vi "Dashboard Main.vi"() -> ()   [LabVIEW 2013]
uses:
  Robot Code - Final/2014 Target Detection/TargetType.ctl
  <vilib>/event_ctls.llb/eventvkey.ctl
  <vilib>/Rock Robotics/WPI/Dashboard/WPI_DashboardLogging Global.vi
  <vilib>/Utility/config.llb/Write Key (String).vi
  <vilib>/Utility/config.llb/Write Key (I32).vi
  <vilib>/Utility/config.llb/NI_LVConfig.lvlib
panel:
  in  "Camera Type":enum16{"206", "1011", "1013"}(ring)=enum."1013"
  out "Image Message":string="Timeout in Camera Communications"
  in  "Rec Mode":enum32{"Stop", "Record", "Playback"}(radio)
  in  "Dashboard Tab":T1(tab)
  in  "X-box":bool caption="Joystick"
  out "Speed (RPM x1000)":dbl(knob) scale=0.0..6.0
  out "Bag Motors":dbl(knob) scale=-1.0..1.0
  out "ENG":bool
  out "DIS":bool
  out "Pickup":dbl(knob) scale=-1.0..1.0 scale format="%#_1g"
  out "Fire":bool
  out "Pick up":bool
  out "Shooter":bool
  in  "Camera Settings":T2={"Frame Rate"=30, "Compression"=30, "Size"=1} {"Frame Rate" scale=1.0..30.0; "Size" items=["640x480", "320x240", "160x120"]}
  out "MotorSliders R":cluster{"MotorSlide1":dbl, "MotorSlide2":dbl} {"MotorSlide2" scale=-1.0..1.0 scale format="%#_2e"; "MotorSlide1" scale=-1.0..1.0 scale format="%#_2e"}
  out "MotorChart R":cluster{"Numeric":dbl, "Numeric":dbl}(graph)
  out "MotorSliders L":T3 {"MotorSlide4 2" scale=0.0..14.0 scale format="%#_2e"; "MotorSlide2" scale=-1.0..1.0 scale format="%#_2e"; "MotorSlide1" scale=-1.0..1.0 scale format="%#_2e"}
  out "MotorChart L":T4(graph)
  out "JS1 Z":dbl(slide) scale=-1.0..1.0 scale format="%#_2e"
  out "Joystick 1":cluster{"X":dbl, "Y":dbl}[](graph)
  out "JS Buttons 1":T5
  out "JS2 Z":dbl(slide) scale=-1.0..1.0 scale format="%#_2e"
  out "Joystick 2":cluster{"X":dbl, "Y":dbl}[](graph)
  out "JS Buttons 2":T5
  out "Mode":T6(ring)=enum."Auto Disabled"
  out "Camera IP":string
  in  "DB Camera Config":bool
  out "fps":dbl format="%#.1g"
  out "Mbps":dbl format="%#.1g"
  out "Mbps 2":bool
  out "LED 1":bool
  in  "Score Limit":dbl=70.0
  out "Distance":dbl
  out "Target Locked On":bool
  in  "Slider 1":dbl(slide) scale=0.0..100.0
  out "Goal is hot":bool
  out "Distances":T8(array[cluster])
  in  "Color Components":T9={"Hue"={110.0, 142.0}, "Sat"={138.0, 255.0}, "Val"={139.0, 198.0}} {"Val" scale=0.0..255.0; "Sat" scale=0.0..255.0; "Hue" scale=0.0..255.0 scale format="%#_3g"}
  in  "Checkbox 2":bool
  in  "Checkbox 1":bool
  in  "Test Slider":dbl(slide) scale=0.0..100.0 scale format="%#_3g"
  in  "On/Off":bool caption="Solenoid"
  in  "Test Name":u16(ring) items=["Select the test to run...", "Example Test", "-------------------------------", "List of tests is built in robot code.", "Replace with your own automated tests."]
  in  "Test Tree":string(tree)
  in  "Motor":cluster{"Value":dbl, "Enable":bool} {"Value" scale=-1.0..1.0 scale format="%#_3g"}
  out "Progress":T10 {"Test Progress" scale=0.0..100.0}
  in  "Rev/Fwd":cluster{"Forward":bool, "Reverse":bool}
  in  "Test Ring":u16(ring) items=["Auto", "Fixed indoor", "Fixed outdoor 1", "Fixed outdoor 2", "Fixed fluorescent 1", "Fixed fluorescent 2", "Hold current"]
  in  "Listbox":i32(listbox)
  out "Tree":string(tree)
  out "Camera Image":T11(plugin-control)
  in  "Enable":bool
  # "Left"
  # "Front"
  # "Right"
  # "Gearbox"
  # "Battery"
  # "Customize by placing controls and indicators here and name to\nmatch Dashboard Variables on robot."
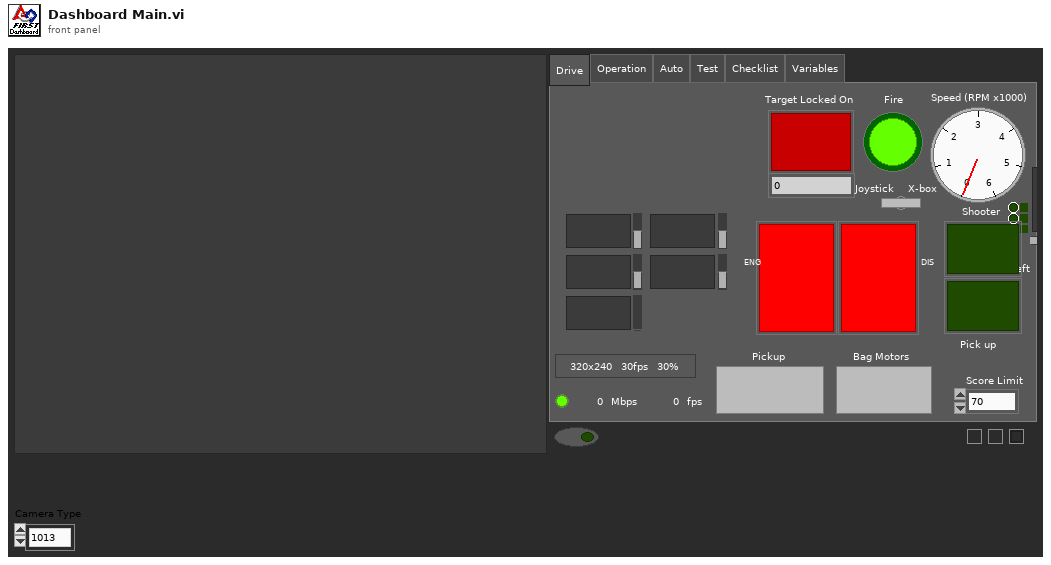
[diagram p1: front panel]
types:
  T1 = enum32{"Drive", "Operation", "Auto", "Test", "Checklist", "Variables"}
  T2 = cluster{"Frame Rate":i32, "Compression":i32, "Size":u16}
  T3 = cluster{"MotorSlide1":dbl, "MotorSlide2":dbl, "MotorSlide4 2":dbl}
  T4 = cluster{"Numeric":dbl, "Numeric":dbl, "Battery":sgl}
  T5 = cluster{bool, bool, bool, bool, bool, bool, bool, bool, bool, bool, bool, bool}
  T6 = enum8{"Tele-Op Disabled", "Tele-Op Enabled", "Auto Disabled", "Auto Enabled", "Test Disabled", "Test Enabled", ""}
  T7 = typedef "TargetType.ctl" = enum16{"Not Hot", "Hot"}
  T8 = cluster{"Distance (ft)":dbl, "Target Center (-1 to 1)":cluster{"X":dbl, "Y":dbl}, "Left":bool, "State":T7}[]
  T9 = cluster{"Hue":cluster{dbl, dbl}, "Sat":cluster{dbl, dbl}, "Val":cluster{dbl, dbl}}
  T10 = cluster{"Test Progress":u8, "Test Progress Text":string}
  T11 = typedef "IMAQ Image.ctl" = refnum<image>
  T12 = typedef "Image Type" = u32
  T13 = cluster{"Digital Inputs":bool[], "Digital Outputs":bool[]}
  T14 = cluster{"Competition mode":bool, "Robot Link":bool, "Autonomous":bool, "Enabled":bool, "E-Stop":bool, "Simulated":bool, "TestMode":bool, "Docked Window":bool}
  T15 = cluster{"Boolean Array[0]":bool, "Boolean Array[1]":bool, "Boolean Array[2]":bool, "Boolean Array[3]":bool, "Boolean Array[4]":bool, "Boolean Array[5]":bool, "Boolean Array[6]":bool, "Boolean Array[7]":bool, "Boolean Array[8]":bool, "Boolean Array[9]":bool, "Boolean Array[10]":bool, "Boolean Array[11]":bool}
  T16 = cluster{"Horizontal":bool, "Aspect Score":dbl, "Rect Score":dbl, cluster{"Left":dbl, "Top":dbl, "Right":dbl, "Bottom":dbl}, "Equiv H":dbl, "Equiv V":dbl}[]
  T17 = cluster{"Scores":cluster{"Total":dbl, "Left":dbl, "Right":dbl, "Ratio":dbl, "Vertical":dbl, "index":i32, "State":T7}, "Verticals":cluster{"Horizontal?":bool, "Aspect Score":dbl, "Rect Score":dbl, cluster{"Left":dbl, "Top":dbl, "Right":dbl, "Bottom":dbl}, "Equiv H":dbl, "Equiv V":dbl}, "Horizontals":cluster{"Horizontal?":bool, "Aspect Score":dbl, "Rect Score":dbl, cluster{"Left":dbl, "Top":dbl, "Right":dbl, "Bottom":dbl}, "Equiv H":dbl, "Equiv V":dbl}, "Validated":bool}[]
  T18 = cluster{"Scores":cluster{"Total":dbl, "Left":dbl, "Right":dbl, "Ratio":dbl, "Vertical":dbl, "index":i32, "State":T7}, "Verticals":cluster{"Horizontal?":bool, "Aspect Score":dbl, "Rect Score":dbl, cluster{"Left":dbl, "Top":dbl, "Right":dbl, "Bottom":dbl}, "Equiv H":dbl, "Equiv V":dbl}, "Horizontals":cluster{"Horizontal?":bool, "Aspect Score":dbl, "Rect Score":dbl, cluster{"Left":dbl, "Top":dbl, "Right":dbl, "Bottom":dbl}, "Equiv H":dbl, "Equiv V":dbl}, "Distance (ft)":dbl, "Target Center (-1 to 1)":cluster{"X":dbl, "Y":dbl}}[]
  T19 = cluster{"Target Info[0]":cluster{"Scores":cluster{"Total":dbl, "Left":dbl, "Right":dbl, "Ratio":dbl, "Vertical":dbl, "index":i32, "State":T7}, "Verticals":cluster{"Horizontal?":bool, "Aspect Score":dbl, "Rect Score":dbl, cluster{"Left":dbl, "Top":dbl, "Right":dbl, "Bottom":dbl}, "Equiv H":dbl, "Equiv V":dbl}, "Horizontals":cluster{"Horizontal?":bool, "Aspect Score":dbl, "Rect Score":dbl, cluster{"Left":dbl, "Top":dbl, "Right":dbl, "Bottom":dbl}, "Equiv H":dbl, "Equiv V":dbl}, "Distance (ft)":dbl, "Target Center (-1 to 1)":cluster{"X":dbl, "Y":dbl}}, "Target Info[1]":cluster{"Scores":cluster{"Total":dbl, "Left":dbl, "Right":dbl, "Ratio":dbl, "Vertical":dbl, "index":i32, "State":T7}, "Verticals":cluster{"Horizontal?":bool, "Aspect Score":dbl, "Rect Score":dbl, cluster{"Left":dbl, "Top":dbl, "Right":dbl, "Bottom":dbl}, "Equiv H":dbl, "Equiv V":dbl}, "Horizontals":cluster{"Horizontal?":bool, "Aspect Score":dbl, "Rect Score":dbl, cluster{"Left":dbl, "Top":dbl, "Right":dbl, "Bottom":dbl}, "Equiv H":dbl, "Equiv V":dbl}, "Distance (ft)":dbl, "Target Center (-1 to 1)":cluster{"X":dbl, "Y":dbl}}, "Target Info[2]":cluster{"Scores":cluster{"Total":dbl, "Left":dbl, "Right":dbl, "Ratio":dbl, "Vertical":dbl, "index":i32, "State":T7}, "Verticals":cluster{"Horizontal?":bool, "Aspect Score":dbl, "Rect Score":dbl, cluster{"Left":dbl, "Top":dbl, "Right":dbl, "Bottom":dbl}, "Equiv H":dbl, "Equiv V":dbl}, "Horizontals":cluster{"Horizontal?":bool, "Aspect Score":dbl, "Rect Score":dbl, cluster{"Left":dbl, "Top":dbl, "Right":dbl, "Bottom":dbl}, "Equiv H":dbl, "Equiv V":dbl}, "Distance (ft)":dbl, "Target Center (-1 to 1)":cluster{"X":dbl, "Y":dbl}}, "Target Info[3]":cluster{"Scores":cluster{"Total":dbl, "Left":dbl, "Right":dbl, "Ratio":dbl, "Vertical":dbl, "index":i32, "State":T7}, "Verticals":cluster{"Horizontal?":bool, "Aspect Score":dbl, "Rect Score":dbl, cluster{"Left":dbl, "Top":dbl, "Right":dbl, "Bottom":dbl}, "Equiv H":dbl, "Equiv V":dbl}, "Horizontals":cluster{"Horizontal?":bool, "Aspect Score":dbl, "Rect Score":dbl, cluster{"Left":dbl, "Top":dbl, "Right":dbl, "Bottom":dbl}, "Equiv H":dbl, "Equiv V":dbl}, "Distance (ft)":dbl, "Target Center (-1 to 1)":cluster{"X":dbl, "Y":dbl}}, "Target Info[4]":cluster{"Scores":cluster{"Total":dbl, "Left":dbl, "Right":dbl, "Ratio":dbl, "Vertical":dbl, "index":i32, "State":T7}, "Verticals":cluster{"Horizontal?":bool, "Aspect Score":dbl, "Rect Score":dbl, cluster{"Left":dbl, "Top":dbl, "Right":dbl, "Bottom":dbl}, "Equiv H":dbl, "Equiv V":dbl}, "Horizontals":cluster{"Horizontal?":bool, "Aspect Score":dbl, "Rect Score":dbl, cluster{"Left":dbl, "Top":dbl, "Right":dbl, "Bottom":dbl}, "Equiv H":dbl, "Equiv V":dbl}, "Distance (ft)":dbl, "Target Center (-1 to 1)":cluster{"X":dbl, "Y":dbl}}, "Target Info[5]":cluster{"Scores":cluster{"Total":dbl, "Left":dbl, "Right":dbl, "Ratio":dbl, "Vertical":dbl, "index":i32, "State":T7}, "Verticals":cluster{"Horizontal?":bool, "Aspect Score":dbl, "Rect Score":dbl, cluster{"Left":dbl, "Top":dbl, "Right":dbl, "Bottom":dbl}, "Equiv H":dbl, "Equiv V":dbl}, "Horizontals":cluster{"Horizontal?":bool, "Aspect Score":dbl, "Rect Score":dbl, cluster{"Left":dbl, "Top":dbl, "Right":dbl, "Bottom":dbl}, "Equiv H":dbl, "Equiv V":dbl}, "Distance (ft)":dbl, "Target Center (-1 to 1)":cluster{"X":dbl, "Y":dbl}}, "Target Info[6]":cluster{"Scores":cluster{"Total":dbl, "Left":dbl, "Right":dbl, "Ratio":dbl, "Vertical":dbl, "index":i32, "State":T7}, "Verticals":cluster{"Horizontal?":bool, "Aspect Score":dbl, "Rect Score":dbl, cluster{"Left":dbl, "Top":dbl, "Right":dbl, "Bottom":dbl}, "Equiv H":dbl, "Equiv V":dbl}, "Horizontals":cluster{"Horizontal?":bool, "Aspect Score":dbl, "Rect Score":dbl, cluster{"Left":dbl, "Top":dbl, "Right":dbl, "Bottom":dbl}, "Equiv H":dbl, "Equiv V":dbl}, "Distance (ft)":dbl, "Target Center (-1 to 1)":cluster{"X":dbl, "Y":dbl}}, "Target Info[7]":cluster{"Scores":cluster{"Total":dbl, "Left":dbl, "Right":dbl, "Ratio":dbl, "Vertical":dbl, "index":i32, "State":T7}, "Verticals":cluster{"Horizontal?":bool, "Aspect Score":dbl, "Rect Score":dbl, cluster{"Left":dbl, "Top":dbl, "Right":dbl, "Bottom":dbl}, "Equiv H":dbl, "Equiv V":dbl}, "Horizontals":cluster{"Horizontal?":bool, "Aspect Score":dbl, "Rect Score":dbl, cluster{"Left":dbl, "Top":dbl, "Right":dbl, "Bottom":dbl}, "Equiv H":dbl, "Equiv V":dbl}, "Distance (ft)":dbl, "Target Center (-1 to 1)":cluster{"X":dbl, "Y":dbl}}, "Target Info[8]":cluster{"Scores":cluster{"Total":dbl, "Left":dbl, "Right":dbl, "Ratio":dbl, "Vertical":dbl, "index":i32, "State":T7}, "Verticals":cluster{"Horizontal?":bool, "Aspect Score":dbl, "Rect Score":dbl, cluster{"Left":dbl, "Top":dbl, "Right":dbl, "Bottom":dbl}, "Equiv H":dbl, "Equiv V":dbl}, "Horizontals":cluster{"Horizontal?":bool, "Aspect Score":dbl, "Rect Score":dbl, cluster{"Left":dbl, "Top":dbl, "Right":dbl, "Bottom":dbl}, "Equiv H":dbl, "Equiv V":dbl}, "Distance (ft)":dbl, "Target Center (-1 to 1)":cluster{"X":dbl, "Y":dbl}}}
  T20 = cluster{cluster{dbl, dbl}, cluster{dbl, dbl}, cluster{dbl, dbl}}
  T21 = typedef "NI_LVConfig.lvlib/Config Data RefNum.ctl" = refnum<k1>
  T22 = typedef "eventvkey.ctl" = enum16{"ASCII", "Enter", "Return", "Shift", "Ctrl", "Alt", "Cmd", "Opt", "Caps", "NumLock", "Clear", "Break", "Up", "Down", "Left", "Right", "Insert", "Delete", "Home", "End", "PageUp", "PageDown", "Escape", "Help", "Pause", "ScrollLock", "F1", "F2", "F3", "F4", "F5", "F6", "F7", "F8", "F9", "F10", "F11", "F12", "F13", "F14", "F15", "F16", "F17", "F18", "F19", "F20", "F21", "F22", "F23", "F24", "Play", "VolumeUp", "VolumeDown", "Mute", "Two Byte Char"}
  T23 = cluster{"Image Size":bool, "Image Type":bool, "Pixel Value":bool, "ROI Information":bool, "Zoom Factor":bool}
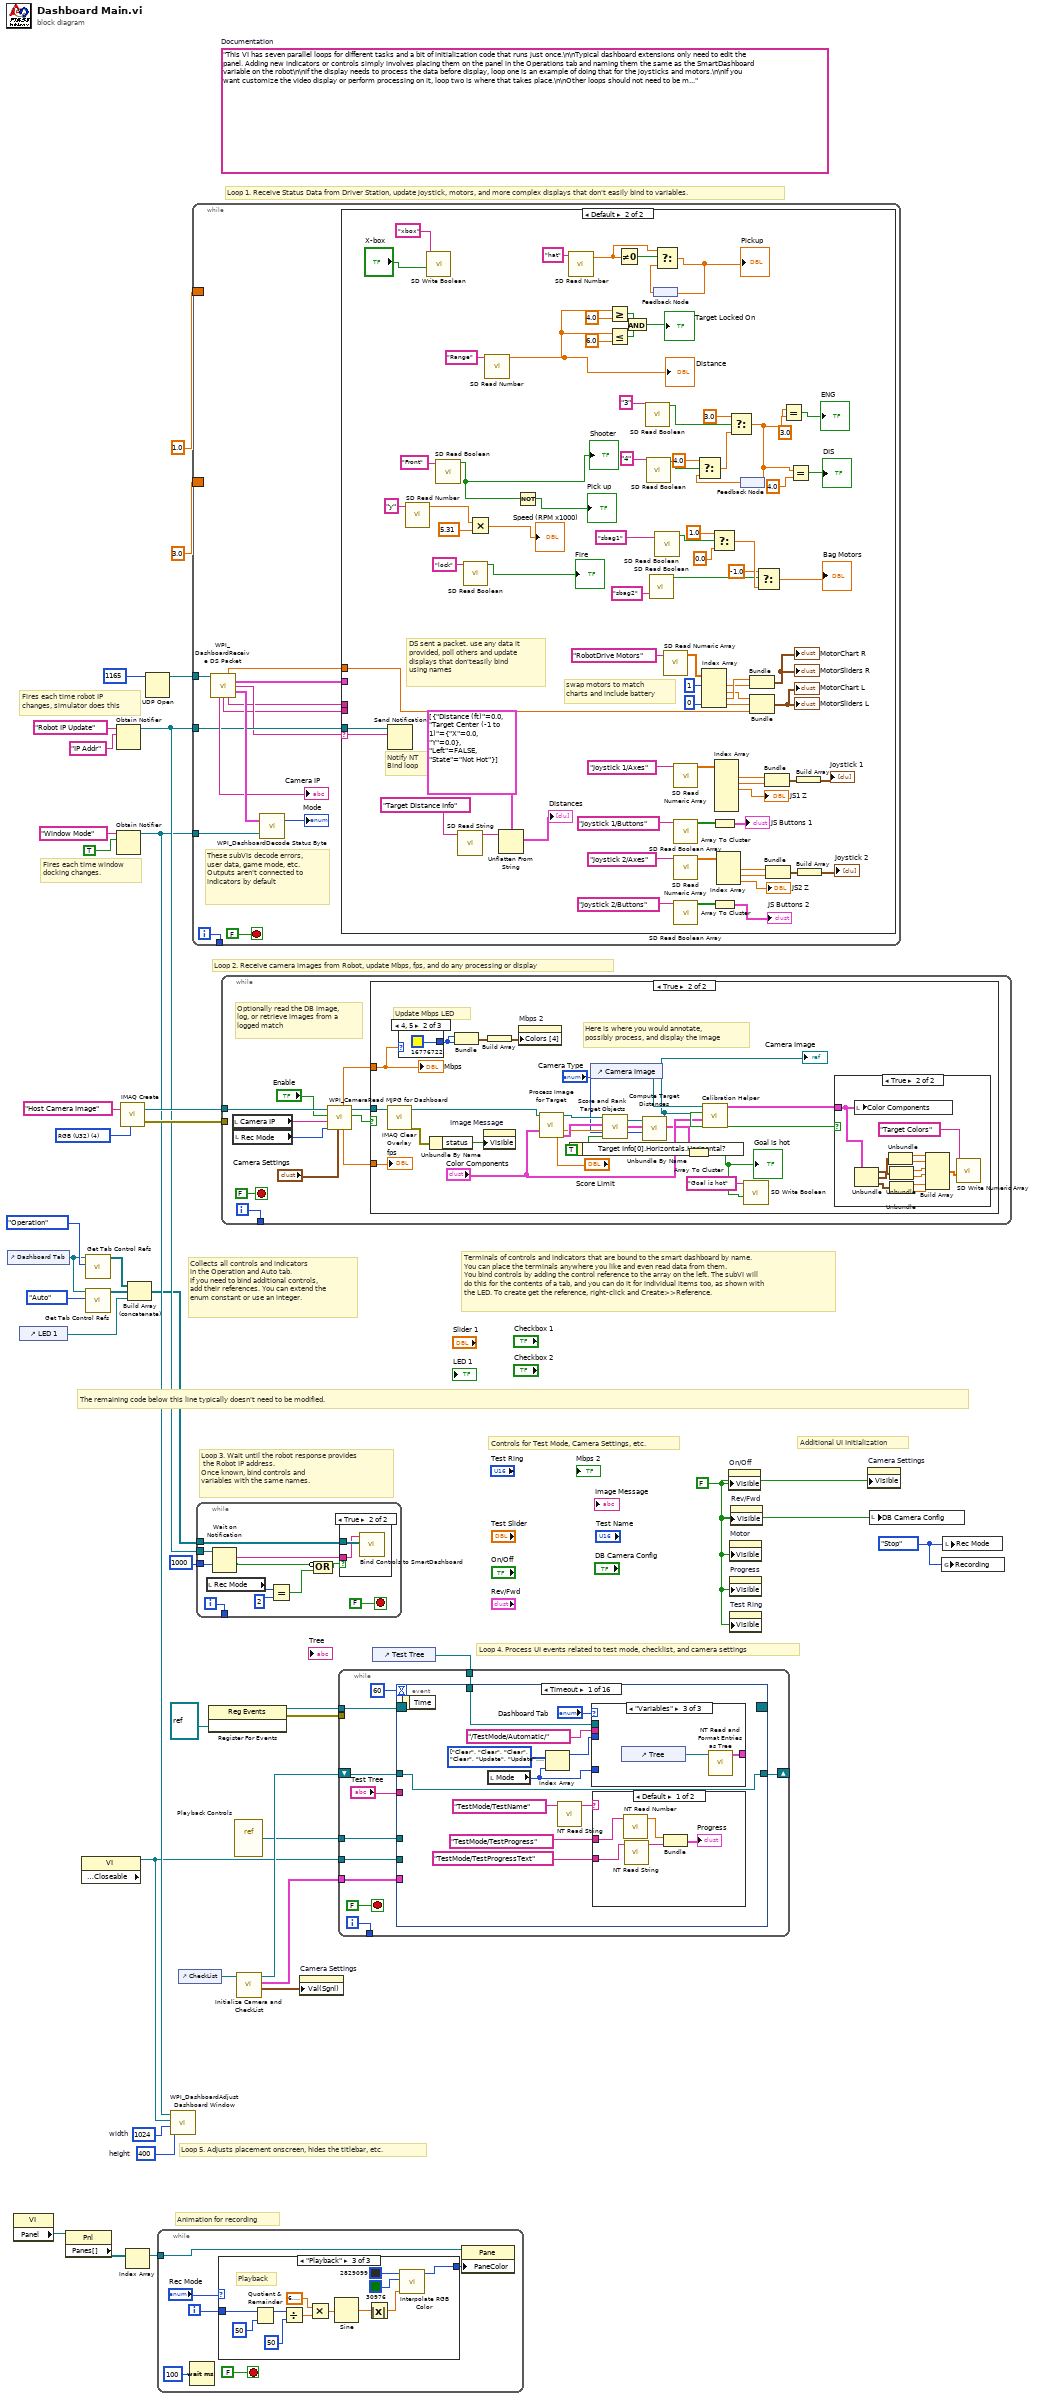
[diagram p0: block diagram]
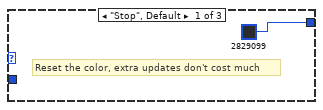
[diagram p2: hidden frame]
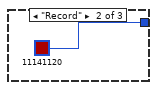
[diagram p3: hidden frame]
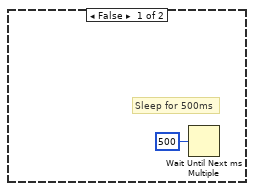
[diagram p5: hidden frame]
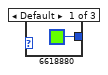
[diagram p7: hidden frame]
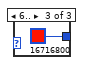
[diagram p8: hidden frame]
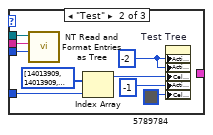
[diagram p10: hidden frame]
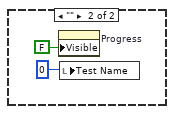
[diagram p11: hidden frame]
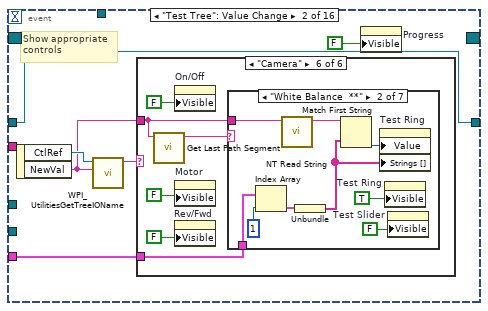
[diagram p12: hidden frame]
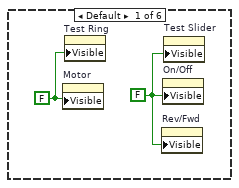
[diagram p13: hidden frame]
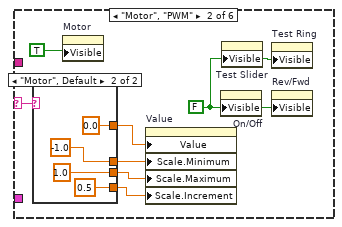
[diagram p14: hidden frame]
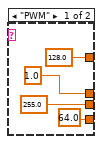
[diagram p15: hidden frame]
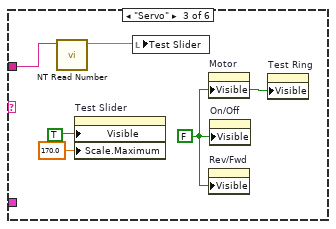
[diagram p16: hidden frame]
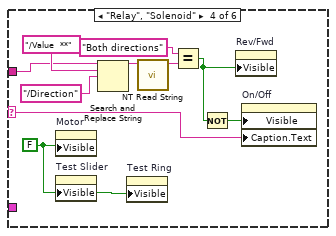
[diagram p17: hidden frame]
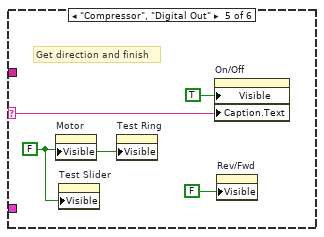
[diagram p18: hidden frame]
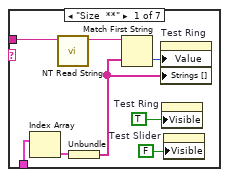
[diagram p19: hidden frame]
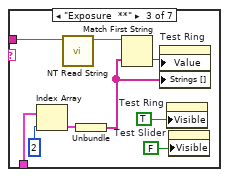
[diagram p20: hidden frame]
diagram:
  w10 = enum32{"Stop", "Record", "Playback"}."Stop" ("Rec Mode")
  w13 = 400  # height
  w14 = 1024  # width
  w27 = FALSE ("Visible")
  (unwired) "This VI has seven parallel loops for different tasks and a bit of initialization code that runs just once.\n\nTypical dashboard extensions only need to edit the panel. Adding new indicators or controls simply involves placing them on the panel in the Operations tab and naming them the same as the SmartDashboard variable on the robot\n\nIf the display needs to process the data before display, loop one is an example of doing that for the joysticks and motors.\n\nIf you want customize the video display or perform processing on it, loop two is where that takes place.\n\nOther loops should not need to be modified. They are pretty standard, and document the task they perform."  # Documentation
  w37 = T12 4 items=["Grayscale (U8)", "Grayscale (I16)", "Grayscale (SGL)", "Complex (CSG)", "RGB (U32)", "HSL (U32)", "RGB (U64)"] ("Image Type")
  # "Controls for Test Mode, Camera Settings, etc."
  # "Additional UI Initialization"
  # "Animation for recording"
  # "Fires each time robot IP\nchanges, simulator does this"
  # "Fires each time window\ndocking changes."
  # "Collects all controls and indicators\nin the Operation and Auto tab.\nIf you need to bind additional controls,\nadd their references. You can extend the\nenum constant or use an integer."
  # "The remaining code below this line typically doesn't need to be modified."
  # "Loop 4. Process UI events related to test mode, checklist, and camera settings"
  # "Terminals of controls and indicators that are bound to the smart dashboard by name.\nYou can place the terminals anywhere you like and even read data from them.\nYou bind controls by adding the control reference to the array on the left. The subVI will\ndo this for the contents of a tab, and you can do it for individual items too, as shown with\nthe LED. To create get the reference, right-click and Create>>Reference."
  # "Loop 3. Wait until the robot response provides\n the Robot IP address.\nOnce known, bind controls and\nvariables with the same names."
  # "Loop 5. Adjusts placement onscreen, hides the titlebar, etc."
  # "Loop 1. Receive Status Data from Driver Station, update joystick, motors, and more complex displays that don't easily bind to variables."
  # "Loop 2. Receive camera images from Robot, update Mbps, fps, and do any processing or display"
  n1 = control-ref of="Dashboard Tab"() -> (w8:refnum<vi>)
  n2 = property class="VI"() -> ("Panel"=w21:refnum<vi>)  [unwired: 2 in, 2 out]
  n3 = control-ref of="LED 1"() -> (w3:refnum<vi>)
  n4 = property class="Pnl"(reference=w21) -> ("Panes[]"=w22:refnum<vi>[])  [unwired: 1 in, 2 out]
  n5 = property class="VI" props=["Front Panel.Closeable"]() -> (reference out=w9:refnum<vi>)  [unwired: 2 in, 2 out]
  n6 = call <vilib>:"Get Tab Control Refs.vi"("Page Index"=T1."Operation" ("Dashboard Tab"), "TabControl in"=w8) -> ("ControlsOnPage"=w6:refnum<vi>[])  [unwired: 9 in]
  n7 = call <vilib>:"Get Tab Control Refs.vi"("Page Index"=T1."Auto" ("Dashboard Tab"), "TabControl in"=w8) -> ("ControlsOnPage"=w7:refnum<vi>[])  [unwired: 9 in]
  n8 = Obtain Notifier(name (unnamed)="Robot IP Update", notification data type="IP Addr" ("name (unnamed)")) -> (notifier out=w31:refnum<notifier>)  [unwired: 2 in, 2 out]
  n9 = Obtain Notifier(name (unnamed)="Window Mode", notification data type=TRUE) -> (notifier out=w12:refnum<notifier>)  [unwired: 2 in, 2 out]
  n10 = call "IMAQ Create"("Image Name"="Host Camera Image", "Image Type"=w37) -> ("New Image"=w35:T11, "error out"=w34:errorcluster)  [unwired: 2 in, 1 out]
  n11 = Index Array(array=w22) -> (element=w20:refnum<vi>)  [unwired: 1 in]
  n12 = Build Array (concatenate)(w6, w7, w3) -> (w5:refnum<vi>[])
  n13 = UDP Open(11:u16 1165 ("port")) -> (port=w38:refnum<k16>)  [unwired: 2 in, 4 out]
  n14 = while {
    tunnel: w20 -> [w41]
    i -> [w44]
    stop <- FALSE stop-if-true
    n15 = Wait (ms)(milliseconds to wait=u32 100) -> ()  [unwired: 1 out]
    n16 = case shown="\"Playback\"" "Rec Mode" {
      tunnel: w44 -> [_ _ w59]
      tunnel: [u32 2829099 ("Base Color") u32 11141120 ("Target Color") w48] -> w40
      frame "Stop", Default {
        # "Reset the color, extra updates don't cost much"
      }
      frame "Record" {
      }
      frame "Playback" {
        # "Playback"
        n17 = Quotient & Remainder(x=w59, y=u32 50 ("milliseconds to wait")) -> (x-y*floor(x/y)=w55:u32)  [unwired: 1 out]
        n18 = Divide(x=w55, y=u32 50 ("milliseconds to wait")) -> (x/y=w52:dbl)
        n19 = Multiply(x=6.283185307179586, y=w52) -> (x*y=w57:dbl)
        n20 = Sine(x=w57) -> (sin(x)=w56:dbl)
        n21 = Absolute Value(x=w56) -> (abs(x)=w49:dbl)
        n22 = call "Interpolate RGB Color.vi"("Proportion"=w49, "Target Color"=u32 30976, "Base Color"=u32 2829099) -> ("Result Color"=w48:u32)  [unwired: 8 in]
      }
    }
    n23 = property class="Pane"(reference=w41, "PaneColor"=w40) -> ()  [unwired: 1 in, 2 out]
  }
  n24 = call <vilib>:"WPI_DashboardAdjust Dashboard Window.vi"("height"=w13, "width"=w14, "reference in"=w9, "Notifier in"=w12) -> ()  [unwired: 8 in]
  n25 = control-ref of="CheckList"() -> (w11:refnum<vi>)
  n26 = while {
    tunnel: w38 -> [w70]
    tunnel: w31 -> [w65]
    tunnel: w12 -> [w69]
    tunnel: [w66] -> _
    border: 3.0 -> [_]
    border: 1.0 ("Numeric") -> [_]
    i -> [w66]
    stop <- FALSE stop-if-true
    # "These subVIs decode errors, user data, game mode, etc.\nOutputs aren't connected to indicators by default"
    n27 = call <vilib>:"WPI_DashboardReceive DS Packet.vi"("Recv Socket"=w70) -> ("Battery"=w60:sgl, "Driver Station"=w61:T13, "Robot IP Address"=w64:string, "Status"=w71:T14, "Camera IP Address"=→"Camera IP":string, "Low Priority User Data"=w63:string, "High Priority User Data"=w62:string)  [unwired: 1 in, 7 out]
    n28 = call <vilib>:"WPI_DashboardDecode Status Byte.vi"("Window Mode Notifier"=w69, "Status"=w71) -> ("Mode"=→"Mode":T6)  [unwired: 1 out]
    n29 = case shown="Default" w64 {
      selector: w64 -> [_ w132]
      tunnel: w65 -> [_ w133]
      tunnel: w63 -> [_ _]
      tunnel: w62 -> [_ _]
      tunnel: w61 -> [_ _]
      tunnel: w60 -> [_ w131]
      frame "0.0.0.0" {
        # "DS not sending packets, or no robot exists yet.\nDon't poll the variables"
      }
      frame Default {
        # "Notify NT\nBind loop"
        # "DS sent a packet. use any data it\nprovided, poll others and update\ndisplays that don'teasily bind\nusing names"
        # "swap motors to match\ncharts and include battery"
        n30 = Send Notification(notification=w132, notifier=w133) -> ()  [unwired: 1 in, 2 out]
        n31 = call <vilib>:"SD Read Number.vi"("Name"="y") -> ("Numeric"=w86:dbl)  [unwired: 8 in, 2 out]
        n32 = call <vilib>:"SD Write Boolean.vi"("Boolean"="X-box", "Name"="xbox") -> ()  [unwired: 8 in, 2 out]
        n33 = call <vilib>:"SD Read Boolean.vi"("Name"="Front") -> ("Boolean"=w88:bool)  [unwired: 8 in, 2 out]
        "Shooter" <- w88
        n34 = call <vilib>:"SD Read String.vi"("Name"="Target Distance Info") -> ("String"=w121:string)  [unwired: 8 in, 2 out]
        n35 = call <vilib>:"SD Read Boolean.vi"("Name"="lock") -> ("Boolean"=→"Fire":bool)  [unwired: 8 in, 2 out]
        n36 = Multiply(x=w86, y=5.31) -> (x*y=→"Speed (RPM x1000)":dbl)
        n37 = call <vilib>:"SD Read Number.vi"("Name"="Range") -> ("Numeric"=w116:dbl)  [unwired: 8 in, 2 out]
        "Distance" <- w116
        n38 = Unflatten From String(type=T8 [{"Distance (ft)"=0.0, "Target Center (-1 to 1)"={"X"=0.0, "Y"=0.0}, "Left"=FALSE, "State"=enum."Not Hot"}] ("Distances"), binary string=w121) -> (value=→"Distances":T8)  [unwired: 3 in, 2 out]
        n39 = Not(x=w88) -> (.not. x?=→"Pick up":bool)
        n40 = call <vilib>:"SD Read Number.vi"("Name"="hat") -> ("Numeric"=w92:dbl)  [unwired: 8 in, 2 out]
        n41 = Greater Or Equal?(x=w116, y=4.0) -> (x >= y?=w113:bool)
        n42 = Less Or Equal?(x=w116, y=6.0) -> (x <= y?=w112:bool)
        n43 = Not Equal To 0?(x=w92) -> (x != 0?=w93:bool)
        n44 = And(x=w113, y=w112) -> (x .and. y?=→"Target Locked On":bool)
        n45 = call <vilib>:"SD Read Boolean.vi"("Name"="3") -> ("Boolean"=w103:bool)  [unwired: 8 in, 2 out]
        n46 = call <vilib>:"SD Read Boolean.vi"("Name"="4") -> ("Boolean"=w104:bool)  [unwired: 8 in, 2 out]
        n47 = call <vilib>:"SD Read Boolean.vi"("Name"="sbag2") -> ("Boolean"=w77:bool)  [unwired: 8 in, 2 out]
        n48 = feedback #1() -> (w90:dbl)
        n49 = Select(t=w92, s=w93, f=w90) -> (s? t:f=w91:dbl)
        "Pickup" <- w91
        n50 = feedback-in #1(w91) -> ()
        n51 = call <vilib>:"SD Read Boolean.vi"("Name"="sbag1") -> ("Boolean"=w82:bool)  [unwired: 8 in, 2 out]
        n52 = call <vilib>:"SD Read Numeric Array.vi"("Name"="RobotDrive Motors") -> ("Numeric Array"=w130:dbl[])  [unwired: 8 in, 2 out]
        n53 = call <vilib>:"SD Read Numeric Array.vi"("Name"="Joystick 1/Axes") -> ("Numeric Array"=w149:dbl[])  [unwired: 8 in, 2 out]
        n54 = call <vilib>:"SD Read Boolean Array.vi"("Name"="Joystick 1/Buttons") -> ("Boolean Array"=w151:bool[])  [unwired: 8 in, 2 out]
        n55 = call <vilib>:"SD Read Numeric Array.vi"("Name"="Joystick 2/Axes") -> ("Numeric Array"=w143:dbl[])  [unwired: 8 in, 2 out]
        n56 = call <vilib>:"SD Read Boolean Array.vi"("Name"="Joystick 2/Buttons") -> ("Boolean Array"=w142:bool[])  [unwired: 8 in, 2 out]
        n57 = Index Array(array=w130, index #1=1, index #4=0) -> (element #1=w126:dbl, element #2=w125:dbl, element #3=w127:dbl, element #4=w122:dbl)  [unwired: 2 in]
        n58 = Select(t=1.0, s=w82, f=0.0) -> (s? t:f=w78:dbl)
        n59 = Array To Cluster(array=w151) -> (cluster=→"JS Buttons 1":T15)
        n60 = Array To Cluster(array=w142) -> (cluster=→"JS Buttons 2":T15)
        n61 = Index Array(array=w149) -> (element #1=w146:dbl, element #2=w147:dbl, element #3=→"JS1 Z":dbl)  [unwired: 6 in, 3 out]
        n62 = Index Array(array=w143) -> (element #1=w138:dbl, element #2=w137:dbl, element #3=→"JS2 Z":dbl)  [unwired: 3 in]
        n63 = feedback #2() -> (w101:dbl)
        n64 = Select(t=4.0, s=w104, f=w101) -> (s? t:f=w102:dbl)
        n65 = Select(t=3.0, s=w103, f=w102) -> (s? t:f=w95:dbl)
        n66 = feedback-in #2(w95) -> ()
        n67 = Bundle("Numeric"=w127, "Numeric"=w126) -> (→"MotorChart R" →"MotorSliders R":cluster{"Numeric":dbl, "Numeric":dbl})  [unwired: 1 in]
        n68 = Bundle("Numeric"=w125, "Numeric"=w122, "Battery"=w131) -> (→"MotorChart L" →"MotorSliders L":T4)  [unwired: 1 in]
        n69 = Select(t=-1.0, s=w77, f=w78) -> (s? t:f=→"Bag Motors":dbl)
        n70 = Bundle("Numeric"=w146, "Numeric"=w147) -> (w145:cluster{"Numeric":dbl, "Numeric":dbl})  [unwired: 1 in]
        n71 = Bundle("Numeric"=w138, "Numeric"=w137) -> (w139:cluster{"Numeric":dbl, "Numeric":dbl})  [unwired: 1 in]
        n72 = Equal?(x=w95, y=3.0) -> (x = y?=→"ENG":bool)
        n73 = Equal?(x=w95, y=4.0) -> (x = y?=→"DIS":bool)
        n74 = Build Array(w145) -> (→"Joystick 1":cluster{"Numeric":dbl, "Numeric":dbl}[])
        n75 = Build Array(w139) -> (→"Joystick 2":cluster{"Numeric":dbl, "Numeric":dbl}[])
      }
    }
  }
  n76 = while {
    tunnel: w5 -> [w165]
    tunnel: w31 -> [w163]
    tunnel: [w161] -> _
    tunnel: u32 1000 ("milliseconds to wait") -> [w160]
    i -> [w161]
    stop <- FALSE stop-if-true
    n77 = local read "Rec Mode"() -> (w156:enum32{"Stop", "Record", "Playback"})
    n78 = Wait on Notification(notifier=w163, timeout in ms (-1)=w160) -> (notification=w162:string, timed out?=w158:bool)  [unwired: 2 in, 2 out]
    n79 = Equal?(x=w156, y=u16 2 ("Rec Mode")) -> (x = y?=w157:bool)
    n80 = Compound Arithmetic op=OR(invert w158, w157) -> (w159:bool)
    n81 = case shown="True" w159 {
      tunnel: w165 -> [_ w167]
      tunnel: w162 -> [_ w166]
      frame False {
      }
      frame True {
        n82 = call <vilib>:"Bind Controls to SmartDashboard.vi"("Bound Control Refs"=w167, "Server IP Address"=w166) -> ()  [unwired: 10 in]
      }
    }
  }
  n83 = register-events(refnum<vi> refnum) -> (reference out=w18:refnum<event-registration>, error out=w17:errorcluster)  [unwired: 2 in]
  n84 = while {
    tunnel: w35 -> [w176]
    tunnel: w34 -> [_]
    tunnel: [w177] -> _
    i -> [w177]
    stop <- FALSE stop-if-true
    # "Optionally read the DB image,\nlog, or retrieve images from a\nlogged match"
    n85 = local read "Camera IP"() -> (w169:string)
    n86 = local read "Rec Mode"() -> (w168:enum32{"Stop", "Record", "Playback"})
    n87 = call <vilib>:"WPI_CameraRead MJPG for Dashboard.vi"("Camera Settings"="Camera Settings", "Rec Mode"=w168, "Camera IP"=w169, "Enable"="Enable", "Refnum in"=w176) -> ("Active"=w173:bool, "Refnum out"=w175:T11, "FPS"=w172:dbl, "Bandwidth (Mbps)"=w171:dbl)  [unwired: 3 in]
    n88 = case shown="True" w173 {
      tunnel: w175 -> [_ w199]
      tunnel: w171 -> [_ w198]
      tunnel: w172 -> [_ w197]
      frame False {
        # "Sleep for 500ms"
        n89 = Wait Until Next ms Multiple(millisecond multiple=u32 500) -> ()  [unwired: 1 out]
      }
      frame True {
        # "Here is where you would annotate,\npossibly process, and display the image"
        # "Update Mbps LED"
        n90 = call "IMAQ Clear Overlay"("Image"=w199) -> ("error out"=w203:errorcluster, "Image Out"=w192:T11)  [unwired: 2 in, 7 out]
        n91 = case shown="4, 5" w198 {
          tunnel: [u32 6618880 ("Color Box") u32 16776722 ("Color Box") u32 16716800 ("Color Box")] -> w200
          frame Default {
          }
          frame 4, 5 {
          }
          frame 6.. {
          }
        }
        n92 = Unbundle By Name(w203) -> ("status"=w204:bool)
        n93 = Bundle("Color Box"=w200, "Color Box"=w200) -> (w202:cluster{"Color Box":u32, "Color Box":u32})  [unwired: 1 out]
        n94 = property on="Image Message" class="Str"("Visible"=w204) -> ()  [unwired: 2 in, 2 out]
        n95 = Build Array(w202) -> (w201:cluster{"Color Box":u32, "Color Box":u32}[])
        n96 = property on="Mbps 2" class="Bool (strict)"("Colors [4]"=w201) -> ()  [unwired: 2 in, 2 out]
        n97 = call "Process Image for Target.vi"("Src Image"=w192, "Color Components"="Color Components") -> ("Src Image Out"=w191:T11, "Particles"=w190:T16)  [unwired: 11 in, 1 out]
        n98 = control-ref of="Camera Image"() -> (w196:refnum<vi>)
        n99 = call "Score and Rank Target Objects.vi"("Annotate"=TRUE, "Score Limit"="Score Limit", "Particles"=w190, "Image in"=w191) -> ("Target Info"=w189:T17, "Annotated Image"=w188:T11)  [unwired: 6 in]
        n100 = call "Compute Target Distances.vi"("Camera Type"="Camera Type", "Target Info"=w189, "Image in"=w188) -> ("Target Info"=w183:T18, "Image out"=w187:T11)  [unwired: 6 in, 1 out]
        "Camera Image" <- w187
        n101 = Array To Cluster(array=w183) -> (cluster=w182:T19)
        n102 = Unbundle By Name(w182) -> ("Target Info[0].Horizontals.Horizontal?"=w181:bool)
        "Goal is hot" <- w181
        n103 = call "Calibration Helper.vi"("Color Components"="Color Components", "Image"=w187, "Image Ctl Refnum"=w196) -> ("Changed"=w194:bool, "output color"=w195:T20)  [unwired: 7 in]
        n104 = call <vilib>:"SD Write Boolean.vi"("Boolean"=w181, "Name"="Goal is hot") -> ()  [unwired: 8 in, 2 out]
        n105 = case shown="True" w194 {
          tunnel: w195 -> [_ w216]
          frame False {
          }
          frame True {
            n106 = local write "Color Components"(w216) -> ()
            n107 = Unbundle(w216) -> (w215:cluster{dbl, dbl}, w214:cluster{dbl, dbl}, w213:cluster{dbl, dbl})
            n108 = Unbundle(w215) -> (w212:dbl, w211:dbl)
            n109 = Unbundle(w214) -> (w210:dbl, w209:dbl)
            n110 = Unbundle(w213) -> (w208:dbl, w207:dbl)
            n111 = Build Array(w212, w211, w210, w209, w208, w207) -> (w206:dbl[])
            n112 = call <vilib>:"SD Write Numeric Array.vi"("Numeric Array"=w206, "Name"="Target Colors") -> ()  [unwired: 8 in, 2 out]
          }
        }
        "Mbps" <- w198
        "fps" <- w197
      }
    }
  }
  n113 = vi-ref "Playback Controls.vi"() -> (w19:refnum<vi>)
  n114 = call "Initialize Camera and CheckList.vi"("ListBox in"=w11) -> ("Cluster"=w25:cluster{"value":i32, "value":i32, "index":i32}, "Array"=w26:cluster{string[]}[], "File Refnum"=w24:T21)  [unwired: 8 in]
  n115 = property on="Camera Settings" class="Clust (strict)"("Val(Sgnl)"=w25) -> ()  [unwired: 2 in, 2 out]
  n116 = control-ref of="Test Tree"() -> (w23:refnum<vi>)
  n117 = while {
    tunnel: w26 -> [w227]
    shift-right: [w226] -> _
    shift-left: w24 -> [w225]
    tunnel: [w224] -> _
    tunnel: w23 -> [w223]
    tunnel: w19 -> [w222]
    tunnel: w18 -> [w221]
    tunnel: w17 -> [_]
    tunnel: w9 -> [w220]
    i -> [w224]
    stop <- FALSE stop-if-true
    n118 = event shown="[0] Timeout" {
      selector: w221 -> [_ _ _ _ _ _ _ _ _ _ _ _ _ _ _ _]
      dyn-events: [_ _ _ _ _ _ _ _ _ _ _ _ _ w465 _ _] -> _
      timeout: u32 60 ("milliseconds to wait") -> [_ _ _ _ _ _ _ _ _ _ _ _ _ _ _ _]
      tunnel: w223 -> [w237 _ _ _ _ _ _ _ _ _ _ _ _ _ _ _]
      tunnel: "Test Tree" -> [_ _ _ _ _ _ _ _ w434 w442 w444 w448 w456 _ _ _]
      tunnel: w227 -> [_ w261 _ _ _ _ w398 w428 _ _ _ _ _ _ _ _]
      tunnel: [w231 w260 w359 w364 w372 w384 w397 w421 w433 w440 w443 w447 w455 w467 w481 w482] -> w226
      tunnel: w225 -> [w231 w260 w359 w364 w372 w384 w396 w421 w433 w440 w443 w447 w455 w467 w481 w482]
      tunnel: w222 -> [_ _ _ _ _ _ _ _ _ _ _ _ _ w468 _ w485]
      tunnel: w220 -> [_ _ _ _ _ _ _ _ _ _ _ _ _ w463 _ _]
      event Timeout {
        w236 = enum16{"Update", "Clear"}[] [enum."Clear", enum."Clear", enum."Clear", enum."Clear", enum."Update", enum."Update", enum."Clear"] items=["Update", "Clear"]
        n119 = event-data() -> ()  [unwired: 1 in, 1 out]
        n120 = local read "Mode"() -> (w234:T6)
        n121 = Index Array(array=w236, index=w234) -> (element=w235:enum16{"Update", "Clear"})
        n122 = call <vilib>:"NT Read String.vi"("Name"="TestMode/TestName") -> ("String"=w240:string)  [unwired: 9 in, 1 out]
        n123 = case shown="\"Variables\"" "Dashboard Tab" {
          tunnel: w237 -> [_ w250 _]
          tunnel: "/TestMode/Automatic/" ("Name Pattern") -> [_ w249 _]
          tunnel: w235 -> [_ w248 _]
          tunnel: w234 -> [_ w246 _]
          tunnel: [_ _ w252] -> _
          frame "Operation", Default {
          }
          frame "Test" {
            w245 = -2 ("Active Item:Row Number")
            n124 = call <vilib>:"NT Read and Format Entries as Tree.vi"("Operation"=w248, "Name Pattern"=w249, "Tree Refnum"=w250) -> ()  [unwired: 7 in, 2 out]
            n125 = Index Array(array=u32[] [14013909, 14013909, 14013909, 14013909, 14013909, 16777215, 14013909], index=w246) -> (element=w244:u32)
            n126 = property on="Test Tree" class="Tree (strict)"("Active Item Row Number"=w245, "ActiveColNum"=w245, "CellBG"=w244, "Active Item Row Number"=-1 ("Active Item:Row Number"), "CellBG"=u32 5789784 ("Color Box")) -> ()  [unwired: 2 in, 2 out]
          }
          frame "Variables" {
            n127 = control-ref of="Tree"() -> (w251:refnum<vi>)
            n128 = call <vilib>:"NT Read and Format Entries as Tree.vi"("Tree Refnum"=w251) -> ("Formatted Strings"=w252:cluster{"Name":string, "Value":string}[])  [unwired: 9 in, 1 out]
          }
        }
        n129 = case shown="Default" w240 {
          tunnel: "TestMode/TestProgress" ("Name") -> [w254 _]
          tunnel: "TestMode/TestProgressText" ("Name") -> [w253 _]
          frame Default {
            n130 = call <vilib>:"NT Read Number.vi"("Name"=w254) -> ("Numeric"=w255:dbl)  [unwired: 9 in, 1 out]
            n131 = call <vilib>:"NT Read String.vi"("Name"=w253) -> ("String"=w256:string)  [unwired: 9 in, 1 out]
            n132 = Bundle("Numeric"=w255, "String"=w256) -> (→"Progress":cluster{"Numeric":dbl, "String":string})  [unwired: 1 in]
          }
          frame "" {
            n133 = property on="Progress" class="Clust (strict)"("Visible"=FALSE) -> ()  [unwired: 2 in, 2 out]
            n134 = local write "Test Name"(u16 0) -> ()
          }
        }
      }
      event "Test Tree": Value Change {
        # "Show appropriate\ncontrols"
        n135 = event-data() -> ("CtlRef"=w264:refnum<vi>, "NewVal"=w262:string)  [unwired: 1 in]
        n136 = call <vilib>:"WPI_UtilitiesGetTreeIOName.vi"("NewVal"=w262, "TreeControl in"=w264) -> ("I/O Name"=w265:string)  [unwired: 9 in]
        n137 = case shown="\"Camera\"" w265 {
          selector: w265 -> [_ w272 _ w290 w299 _]
          tunnel: w262 -> [_ _ w287 w289 _ w306]
          tunnel: w261 -> [_ _ _ _ _ w305]
          frame Default {
            w267 = FALSE ("Visible")
            w266 = FALSE ("Visible")
            n138 = property on="Motor" class="Clust (strict)"("Visible"=w266) -> ()  [unwired: 2 in, 2 out]
            n139 = property on="Test Ring" class="Ring (strict)"("Visible"=w266) -> ()  [unwired: 2 in, 2 out]
            n140 = property on="Rev/Fwd" class="Clust (strict)"("Visible"=w267) -> ()  [unwired: 2 in, 2 out]
            n141 = property on="On/Off" class="Bool (strict)"("Visible"=w267) -> ()  [unwired: 2 in, 2 out]
            n142 = property on="Test Slider" class="Slide (strict)"("Visible"=w267) -> ()  [unwired: 2 in, 2 out]
          }
          frame "Motor", "PWM" {
            w273 = FALSE ("Visible")
            n143 = case shown="\"Motor\", Default" w272 {
              tunnel: [1.0 ("Value") -1.0 ("Value")] -> w271
              tunnel: [255.0 ("Value") 1.0 ("Value")] -> w270
              tunnel: [128.0 ("Value") 0.0 ("Value")] -> w269
              tunnel: [64.0 ("Value") 0.5 ("Value")] -> w268
              frame "PWM" {
              }
              frame "Motor", Default {
              }
            }
            n144 = property on="Motor" class="Clust (strict)"("Visible"=TRUE) -> ()  [unwired: 2 in, 2 out]
            n145 = property on="Value" class="Slide (strict)"("Value"=w269, "Scale.Minimum"=w271, "Scale.Maximum"=w270, "Scale.Increment"=w268) -> ()  [unwired: 2 in, 2 out]
            n146 = property on="On/Off" class="Bool (strict)"("Visible"=w273) -> ()  [unwired: 2 in, 2 out]
            n147 = property on="Test Slider" class="Slide (strict)"("Visible"=w273) -> ()  [unwired: 2 in, 2 out]
            n148 = property on="Test Ring" class="Ring (strict)"("Visible"=w273) -> ()  [unwired: 2 in, 2 out]
            n149 = property on="Rev/Fwd" class="Clust (strict)"("Visible"=w273) -> ()  [unwired: 2 in, 2 out]
          }
          frame "Servo" {
            w285 = FALSE ("Visible")
            n150 = call <vilib>:"NT Read Number.vi"("Name"=w287) -> ("Numeric"=w286:dbl)  [unwired: 9 in, 1 out]
            n151 = property on="Test Slider" class="Slide (strict)"("Visible"=TRUE, "Scale.Maximum"=170.0 ("Scale.Range:Maximum")) -> ()  [unwired: 2 in, 2 out]
            n152 = local write "Test Slider"(w286) -> ()
            n153 = property on="Motor" class="Clust (strict)"("Visible"=w285) -> ()  [unwired: 2 in, 2 out]
            n154 = property on="Rev/Fwd" class="Clust (strict)"("Visible"=w285) -> ()  [unwired: 2 in, 2 out]
            n155 = property on="On/Off" class="Bool (strict)"("Visible"=w285) -> ()  [unwired: 2 in, 2 out]
            n156 = property on="Test Ring" class="Ring (strict)"("Visible"=w285) -> ()  [unwired: 2 in, 2 out]
          }
          frame "Relay", "Solenoid" {
            w288 = FALSE ("Visible")
            n157 = property on="Motor" class="Clust (strict)"("Visible"=w288) -> ()  [unwired: 2 in, 2 out]
            n158 = property on="Test Slider" class="Slide (strict)"("Visible"=w288) -> ()  [unwired: 2 in, 2 out]
            n159 = Search and Replace String(input string=w289, search string="/Value  **", replace string="/Direction") -> (result string=w295:string)  [unwired: 5 in, 3 out]
            n160 = property on="Test Ring" class="Ring (strict)"("Visible"=w288) -> ()  [unwired: 2 in, 2 out]
            n161 = call <vilib>:"NT Read String.vi"("Name"=w295) -> ("String"=w293:string)  [unwired: 9 in, 1 out]
            n162 = Equal?(x="Both directions", y=w293) -> (x = y?=w291:bool)
            n163 = Not(x=w291) -> (.not. x?=w292:bool)
            n164 = property on="Rev/Fwd" class="Clust (strict)"("Visible"=w291) -> ()  [unwired: 2 in, 2 out]
            n165 = property on="On/Off" class="Bool (strict)"("Visible"=w292, "Caption.Text"=w290) -> ()  [unwired: 2 in, 2 out]
          }
          frame "Compressor", "Digital Out" {
            w298 = FALSE ("Visible")
            # "Get direction and finish"
            n166 = property on="Motor" class="Clust (strict)"("Visible"=w298) -> ()  [unwired: 2 in, 2 out]
            n167 = property on="Test Slider" class="Slide (strict)"("Visible"=w298) -> ()  [unwired: 2 in, 2 out]
            n168 = property on="Test Ring" class="Ring (strict)"("Visible"=w298) -> ()  [unwired: 2 in, 2 out]
            n169 = property on="On/Off" class="Bool (strict)"("Visible"=TRUE, "Caption.Text"=w299) -> ()  [unwired: 2 in, 2 out]
            n170 = property on="Rev/Fwd" class="Clust (strict)"("Visible"=FALSE) -> ()  [unwired: 2 in, 2 out]
          }
          frame "Camera" {
            n171 = call <vilib>:"Get Last Path Segment.vi"("String in"=w306) -> ("String out"=w307:string)  [unwired: 10 in]
            n172 = property on="On/Off" class="Bool (strict)"("Visible"=FALSE) -> ()  [unwired: 2 in, 2 out]
            n173 = property on="Motor" class="Clust (strict)"("Visible"=FALSE) -> ()  [unwired: 2 in, 2 out]
            n174 = property on="Rev/Fwd" class="Clust (strict)"("Visible"=FALSE) -> ()  [unwired: 2 in, 2 out]
            n175 = case shown="\"White Balance  **\"" w307 {
              tunnel: w306 -> [w313 w322 w331 w340 w349 _ w355]
              tunnel: w305 -> [w311 w319 w328 w337 w346 _ _]
              frame "Size  **" {
                n176 = Index Array(array=w311) -> (element=w310:cluster{string[]})  [unwired: 1 in]
                n177 = call <vilib>:"NT Read String.vi"("Name"=w313) -> ("String"=w312:string)  [unwired: 9 in, 1 out]
                n178 = Unbundle(w310) -> (w308:string[])
                n179 = Match First String(2:w308, 3:w312) -> (0:w309:i32)  [unwired: 1 out]
                n180 = property on="Test Ring" class="Ring (strict)"("Value"=w309, "Strings []"=w308) -> ()  [unwired: 2 in, 2 out]
                n181 = property on="Test Ring" class="Ring (strict)"("Visible"=TRUE) -> ()  [unwired: 2 in, 2 out]
                n182 = property on="Test Slider" class="Slide (strict)"("Visible"=FALSE) -> ()  [unwired: 2 in, 2 out]
              }
              frame "White Balance  **" {
                n183 = Index Array(array=w319, index=1) -> (element=w320:cluster{string[]})
                n184 = call <vilib>:"NT Read String.vi"("Name"=w322) -> ("String"=w321:string)  [unwired: 9 in, 1 out]
                n185 = Unbundle(w320) -> (w317:string[])
                n186 = Match First String(2:w317, 3:w321) -> (0:w316:i32)  [unwired: 1 out]
                n187 = property on="Test Ring" class="Ring (strict)"("Value"=w316, "Strings []"=w317) -> ()  [unwired: 2 in, 2 out]
                n188 = property on="Test Ring" class="Ring (strict)"("Visible"=TRUE) -> ()  [unwired: 2 in, 2 out]
                n189 = property on="Test Slider" class="Slide (strict)"("Visible"=FALSE) -> ()  [unwired: 2 in, 2 out]
              }
              frame "Exposure  **" {
                n190 = Index Array(array=w328, index=2) -> (element=w329:cluster{string[]})
                n191 = call <vilib>:"NT Read String.vi"("Name"=w331) -> ("String"=w330:string)  [unwired: 9 in, 1 out]
                n192 = Unbundle(w329) -> (w325:string[])
                n193 = Match First String(2:w325, 3:w330) -> (0:w326:i32)  [unwired: 1 out]
                n194 = property on="Test Ring" class="Ring (strict)"("Value"=w326, "Strings []"=w325) -> ()  [unwired: 2 in, 2 out]
                n195 = property on="Test Ring" class="Ring (strict)"("Visible"=TRUE) -> ()  [unwired: 2 in, 2 out]
                n196 = property on="Test Slider" class="Slide (strict)"("Visible"=FALSE) -> ()  [unwired: 2 in, 2 out]
              }
              frame "Exposure Priority  **" {
                n197 = Index Array(array=w337, index=3) -> (element=w338:cluster{string[]})
                n198 = call <vilib>:"NT Read String.vi"("Name"=w340) -> ("String"=w339:string)  [unwired: 9 in, 1 out]
                n199 = Unbundle(w338) -> (w334:string[])
                n200 = Match First String(2:w334, 3:w339) -> (0:w335:i32)  [unwired: 1 out]
                n201 = property on="Test Ring" class="Ring (strict)"("Value"=w335, "Strings []"=w334) -> ()  [unwired: 2 in, 2 out]
                n202 = property on="Test Ring" class="Ring (strict)"("Visible"=TRUE) -> ()  [unwired: 2 in, 2 out]
                n203 = property on="Test Slider" class="Slide (strict)"("Visible"=FALSE) -> ()  [unwired: 2 in, 2 out]
              }
              frame "Color Enable  **" {
                n204 = Index Array(array=w346, index=4) -> (element=w347:cluster{string[]})
                n205 = call <vilib>:"NT Read String.vi"("Name"=w349) -> ("String"=w348:string)  [unwired: 9 in, 1 out]
                n206 = Unbundle(w347) -> (w343:string[])
                n207 = Match First String(2:w343, 3:w348) -> (0:w344:i32)  [unwired: 1 out]
                n208 = property on="Test Ring" class="Ring (strict)"("Value"=w344, "Strings []"=w343) -> ()  [unwired: 2 in, 2 out]
                n209 = property on="Test Ring" class="Ring (strict)"("Visible"=TRUE) -> ()  [unwired: 2 in, 2 out]
                n210 = property on="Test Slider" class="Slide (strict)"("Visible"=FALSE) -> ()  [unwired: 2 in, 2 out]
              }
              frame Default {
                n211 = property on="Test Ring" class="Ring (strict)"("Visible"=FALSE) -> ()  [unwired: 2 in, 2 out]
                n212 = property on="Test Slider" class="Slide (strict)"("Visible"=FALSE) -> ()  [unwired: 2 in, 2 out]
              }
              frame "Brightness  **", "Color Level  **", "Compression  **", "FPS  **", "Sharpness  **" {
                n213 = call <vilib>:"NT Read Number.vi"("Name"=w355) -> ("Numeric"=w354:dbl)  [unwired: 9 in, 1 out]
                n214 = local write "Test Slider"(w354) -> ()
                n215 = property on="Test Slider" class="Slide (strict)"("Visible"=TRUE, "Scale.Maximum"=100.0 ("Scale.Range:Maximum")) -> ()  [unwired: 2 in, 2 out]
                n216 = property on="Test Ring" class="Ring (strict)"("Visible"=FALSE) -> ()  [unwired: 2 in, 2 out]
              }
            }
          }
        }
        n217 = property on="Progress" class="Clust (strict)"("Visible"=FALSE) -> ()  [unwired: 2 in, 2 out]
      }
      event "Test Name": Mouse Enter {
        # "Populate the ring with the list of tests"
        n218 = event-data() -> ()  [unwired: 1 in, 1 out]
        n219 = call <vilib>:"NT Read String Array.vi"("Name"="TestMode/TestList") -> ("String Array"=w363:string[])  [unwired: 9 in, 1 out]
        n220 = Build Array (concatenate)("Select the test to run...", w363) -> (w362:string[])
        n221 = property on="Test Name" class="Ring (strict)"("Strings []"=w362) -> ()  [unwired: 2 in, 2 out]
      }
      event "Test Name": Value Change {
        w365 = FALSE ("Visible")
        # "Tell the robot the test name to run"
        n222 = event-data() -> ("NewVal"=w369:u16)  [unwired: 1 in]
        n223 = property on="Test Name" class="Ring (strict)"() -> ("Strings []"=w370:string[])  [unwired: 2 in, 2 out]
        n224 = local write "Progress"(T10 {"Test Progress"=0, "Test Progress Text"=""} ("Progress")) -> ()
        n225 = Index Array(array=w370, index=w369) -> (element=w368:string)
        n226 = call <vilib>:"NT Write String.vi"("String"=w368, "Name"="TestMode/TestName") -> ()  [unwired: 9 in, 1 out]
        n227 = property on="Progress" class="Clust (strict)"("Visible"=TRUE) -> ()  [unwired: 2 in, 2 out]
        n228 = property on="Motor" class="Clust (strict)"("Visible"=w365) -> ()  [unwired: 2 in, 2 out]
        n229 = property on="Test Slider" class="Slide (strict)"("Visible"=w365) -> ()  [unwired: 2 in, 2 out]
        n230 = property on="On/Off" class="Bool (strict)"("Visible"=w365) -> ()  [unwired: 2 in, 2 out]
        n231 = property on="Rev/Fwd" class="Clust (strict)"("Visible"=w365) -> ()  [unwired: 2 in, 2 out]
        n232 = property on="Test Ring" class="Ring (strict)"("Visible"=w365) -> ()  [unwired: 2 in, 2 out]
      }
      event "Listbox": Double Click {
        n233 = event-data() -> ("PlatMods.Shift"=w373:bool, "Row"=w375:i32)  [unwired: 1 in]
        n234 = case shown="True" w373 {
          tunnel: w375 -> [w379 _]
          tunnel: 1 -> [w378 _]
          frame False {
            n235 = property on="Listbox" class="LstBox (strict)"() -> ("Item Symbols"=w377:i32[])  [unwired: 2 in, 2 out]
            n236 = Replace Array Subset(array=w377, new element=w378, index=w379) -> (w376:i32[])
            n237 = property on="Listbox" class="LstBox (strict)"("Item Symbols"=w376) -> ()  [unwired: 2 in, 2 out]
          }
          frame True {
            w380 = 0 ("Top Row")
            n238 = property on="Listbox" class="LstBox (strict)"() -> ("Number of Rows"=w382:u32)  [unwired: 2 in, 2 out]
            n239 = Initialize Array(0, w382) -> (w381:i32[])
            n240 = property on="Listbox" class="LstBox (strict)"("Top Row"=w380, "Value"=w380, "Item Symbols"=w381) -> ()  [unwired: 2 in, 2 out]
          }
        }
      }
      event "Listbox": Key Down {
        n241 = event-data() -> ("VKey"=w386:T22)  [unwired: 1 in]
        n242 = case shown="\"Left\", \"Right\"" w386 {
          selector: w386 -> [w391 _]
          tunnel: eventvkey."Left" ("VKey") -> [w389 _]
          frame "Left", "Right" {
            n243 = Equal?(x=w389, y=w391) -> (x = y?=w390:bool)
            n244 = Select(t=0, s=w390, f=1) -> (s? t:f=w392:i32)
            n245 = property on="Listbox" class="LstBox (strict)"() -> ("Item Symbols"=w395:i32[])  [unwired: 2 in, 2 out]
            n246 = Replace Array Subset(array=w395, new element=w392, index="Listbox") -> (w394:i32[])
            n247 = property on="Listbox" class="LstBox (strict)"("Item Symbols"=w394) -> ()  [unwired: 2 in, 2 out]
          }
          frame Default {
          }
        }
      }
      event "DB Camera Config": Value Change {
        n248 = event-data() -> ("NewVal"=w399:bool)  [unwired: 1 in]
        n249 = case shown="False" w399 {
          tunnel: w398 -> [w408 _]
          tunnel: [w401 w419] -> w397
          tunnel: w396 -> [w400 w419]
          frame False {
            w415 = "Camera"
            w418 = FALSE ("Visible")
            n250 = local read "Camera Settings"() -> (w407:T2)
            n251 = Index Array(array=w408) -> (element=w411:cluster{string[]})  [unwired: 1 in]
            n252 = Unbundle(w407) -> ("Frame Rate"=w406:i32, "Compression"=w405:i32, "Size"=w409:u16)
            n253 = Unbundle(w411) -> (w410:string[])
            n254 = Index Array(array=w410, index=w409) -> (element=w404:string)
            n255 = call-poly <vilib>:"Write Key.vi"("section"=w415, "value"=w404, "key"="Size", "refnum"=w400) -> ("refnum out"=w417:T21)  [unwired: 2 in, 5 out]
            n256 = call-poly <vilib>:"Write Key.vi"("section"=w415, "value"=w406, "key"="FrameRate", "refnum"=w417) -> ("refnum out"=w416:T21)  [unwired: 1 in, 6 out]
            n257 = property on="Camera Settings" class="Clust (strict)"("Visible"=w418) -> ()  [unwired: 2 in, 2 out]
            n258 = local write "DB Camera Config"(w418) -> ()
            n259 = call-poly <vilib>:"Write Key.vi"("section"=w415, "value"=w405, "key"="Compression", "refnum"=w416) -> ("refnum out"=w402:T21)  [unwired: 1 in, 6 out]
            n260 = call <vilib>:"Close Config Data.vi"("refnum"=w402) -> ("file path"=w403:path)  [unwired: 2 in, 8 out]
            n261 = call <vilib>:"Open Config Data.vi"("configuration file path"=w403) -> ("refnum"=w401:T21)  [unwired: 8 in, 2 out]
          }
          frame True {
            n262 = property on="Camera Settings" class="Clust (strict)"("Visible"=TRUE) -> ()  [unwired: 2 in, 2 out]
          }
        }
      }
      event "Camera Settings": Value Change {
        n263 = event-data() -> ("NewVal"=w432:T2)  [unwired: 1 in]
        n264 = Index Array(array=w428) -> (element=w427:cluster{string[]})  [unwired: 1 in]
        n265 = Unbundle(w432) -> ("Frame Rate"=w423:i32, "Compression"=w422:i32, "Size"=w425:u16)
        n266 = Unbundle(w427) -> (w426:string[])
        n267 = Index Array(array=w426, index=w425) -> (element=w424:string)
        n268 = Format Into String(format string="%s   %dfps   %d%%", w424, w423, w422) -> (resulting string=w429:string)  [unwired: 2 in, 1 out]
        n269 = Build Array(w429) -> (w430:string[])
        n270 = property on="DB Camera Config" class="Bool (strict)"("Strings [4]"=w430) -> ()  [unwired: 2 in, 2 out]
      }
      event "Motor.Enable": Value Change {
        n271 = event-data() -> ("NewVal"=w438:bool)  [unwired: 1 in]
        n272 = Unbundle("Motor") -> ("Value"=w437:dbl)  [unwired: 1 out]
        n273 = Select(t=w437, s=w438, f=0.0) -> (s? t:f=w435:dbl)
        n274 = call <vilib>:"NT Write Number.vi"("Numeric"=w435, "Name"=w434) -> ()  [unwired: 9 in, 1 out]
      }
      event "Test Slider": Value Change {
        n275 = event-data() -> ("NewVal"=w441:dbl)  [unwired: 1 in]
        n276 = call <vilib>:"NT Write Number.vi"("Numeric"=w441, "Name"=w442) -> ()  [unwired: 9 in, 1 out]
      }
      event "On/Off": Value Change {
        n277 = event-data() -> ("NewVal"=w446:bool)  [unwired: 1 in]
        n278 = Boolean To (0,1)(Boolean=w446) -> (0, 1=w445:i16)
        n279 = call <vilib>:"NT Write Number.vi"("Numeric"=w445, "Name"=w444) -> ()  [unwired: 9 in, 1 out]
      }
      event "Rev/Fwd": Value Change {
        n280 = event-data() -> ("NewVal.Forward"=w454:bool, "NewVal.Reverse"=w453:bool)  [unwired: 1 in]
        n281 = Boolean To (0,1)(Boolean=w454) -> (0, 1=w450:i16)
        n282 = Boolean To (0,1)(Boolean=w453) -> (0, 1=w452:i16)
        n283 = Negate(x=w452) -> (-x=w451:i16)
        n284 = Add(x=w450, y=w451) -> (x+y=w449:i16)
        n285 = call <vilib>:"NT Write Number.vi"("Numeric"=w449, "Name"=w448) -> ()  [unwired: 9 in, 1 out]
      }
      event "Test Ring": Value Change {
        n286 = event-data() -> ("NewVal"=w458:u16)  [unwired: 1 in]
        n287 = property on="Test Ring" class="Ring (strict)"() -> ("Strings []"=w459:string[])  [unwired: 2 in, 2 out]
        n288 = Index Array(array=w459, index=w458) -> (element=w457:string)
        n289 = call <vilib>:"NT Write String.vi"("String"=w457, "Name"=w456) -> ()  [unwired: 9 in, 1 out]
      }
      event "Rec Mode": Value Change {
        # "Update globals for recording mode and path to read log from.\nClear when logging and let NetworkTables set path for vision to\nuse."
        n290 = event-data() -> ("NewVal"=w469:enum32{"Stop", "Record", "Playback"})  [unwired: 1 in]
        n291 = global write "WPI_DashboardLogging Global.vi" "Logging Filename"(path "") -> ()
        n292 = case shown="\"Stop\", \"Record\"" w469 {
          tunnel: w468 -> [_ w471 w479]
          tunnel: [_ _ w478] -> w465
          tunnel: [_ _ w477] -> _
          tunnel: w463 -> [_ _ w475]
          tunnel: cluster{i32, i32} {-250, 170} -> [_ _ w474]
          tunnel: [_ _ T23 {"Image Size"=TRUE, "Image Type"=TRUE, "Pixel Value"=TRUE, "ROI Information"=TRUE, "Zoom Factor"=FALSE} ("Image Information Shown:All Elements")] -> w461
          tunnel: [_ _ TRUE ("Zoom Factor")] -> w460
          frame Default {
          }
          frame "Stop", "Record" {
            # "Place Window too"
            n293 = invoke class="VI" method="FP.Close"(reference=w471) -> (reference out=w470:refnum<vi>)  [unwired: 2 in, 2 out]
            n294 = invoke class="VI" method="Abort VI"(reference=w470) -> ()  [unwired: 2 in, 3 out]
          }
          frame "Playback" {
            n295 = call "Open Playback Panel.vi"("Offset"=w474, "DB VI Ref"=w475, "Playback in"=w479) -> ("Playback out"=w476:refnum<vi>)  [unwired: 8 in]
            n296 = register-events(w476) -> (reference out=w478:refnum<event-registration>, error out=w477:errorcluster)  [unwired: 2 in]
          }
        }
        n297 = global write "WPI_DashboardLogging Global.vi" "Recording"(w469) -> ()
        n298 = property on="Camera Image" class="ImageControl"("Image Information Shown"=w461, "Image Information Visible"=w460) -> ()  [unwired: 2 in, 2 out]
        n299 = call <vilib>:"WPI_DashboardNT Log FieldName Cache.vi"("Operation"=enum16{"Lookup/Add", "Index", "Clear"}."Clear") -> ()  [unwired: 8 in, 3 out]
      }
      event Panel Close {
        w480 = enum32{"Stop", "Record", "Playback"}."Stop" ("Rec Mode")
        n300 = event-data() -> ()  [unwired: 1 in, 4 out]
        n301 = local write "Rec Mode"(w480) -> ()
        n302 = global write "WPI_DashboardLogging Global.vi" "Recording"(w480) -> ()
      }
      event Panel Close {
        # "Abort playback window and ourself"
        n303 = event-data() -> ()  [unwired: 1 in, 4 out]
        n304 = invoke class="VI" method="FP.Close"(reference=w485) -> (reference out=w484:refnum<vi>)  [unwired: 2 in, 2 out]
        n305 = invoke class="VI" method="Abort VI"(reference=w484) -> (error out=w483:errorcluster)  [unwired: 2 in, 2 out]
        n306 = invoke class="VI" method="Abort VI"(error in=w483) -> ()  [unwired: 2 in, 3 out]
      }
    }
  }
  n307 = property on="On/Off" class="Bool (strict)"("Visible"=w27) -> ()  [unwired: 2 in, 2 out]
  n308 = property on="Motor" class="Clust (strict)"("Visible"=w27) -> ()  [unwired: 2 in, 2 out]
  n309 = property on="Progress" class="Clust (strict)"("Visible"=w27) -> ()  [unwired: 2 in, 2 out]
  n310 = property on="Test Ring" class="Ring (strict)"("Visible"=w27) -> ()  [unwired: 2 in, 2 out]
  n311 = property on="Rev/Fwd" class="Clust (strict)"("Visible"=w27) -> ()  [unwired: 2 in, 2 out]
  n312 = property on="Camera Settings" class="Clust (strict)"("Visible"=w27) -> ()  [unwired: 2 in, 2 out]
  n313 = local write "DB Camera Config"(w27) -> ()
  n314 = global write "WPI_DashboardLogging Global.vi" "Recording"(w10) -> ()
  n315 = local write "Rec Mode"(w10) -> ()
